vi "M14_Intake_Hardware_Globals.vi"() -> ()   [LabVIEW 2019]
panel:
  in  "Intake Motor A":string
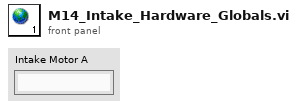
[diagram p1: front panel]
diagram:
